vi "MV3D RGBD Set Param.vi"(9 "pstParam":T1={"enParamType"=1, "nReserved[0]"=0, "nReserved[1]"=0, "nReserved[2]"=0, "nReserved[3]"=0, "nReserved[4]"=0, "nReserved[5]"=0, "nReserved[6]"=0, "nReserved[7]"=0, "nReserved[8]"=0, "nReserved[9]"=0, "nReserved[10]"=0, "nReserved[11]"=0, "nReserved[12]"=0, "nReserved[13]"=0, "nReserved[14]"=0, "nReserved[15]"=0} {"enParamType" items=["ParamType_Bool"=1, "ParamType_Int"=2, "ParamType_Float"=3, "ParamType_Enum"=4, "ParamType_String"=5]}, 10 "strKey":string, 11 "handle":u32) -> (1 "pstParam out":T1={"enParamType"=1, "nReserved[0]"=0, "nReserved[1]"=0, "nReserved[2]"=0, "nReserved[3]"=0, "nReserved[4]"=0, "nReserved[5]"=0, "nReserved[6]"=0, "nReserved[7]"=0, "nReserved[8]"=0, "nReserved[9]"=0, "nReserved[10]"=0, "nReserved[11]"=0, "nReserved[12]"=0, "nReserved[13]"=0, "nReserved[14]"=0, "nReserved[15]"=0} {"enParamType" items=["ParamType_Bool"=1, "ParamType_Int"=2, "ParamType_Float"=3, "ParamType_Enum"=4, "ParamType_String"=5]}, 2 "function return":i32, 3 "handle out":u32)   [LabVIEW 2015, in "Mv3dRgbd.lvlib"]
doc: "MV3D_RGBD_API MV3D_RGBD_STATUS MV3D_RGBD_SetParam(HANDLE handle, const char* strKey, MV3D_RGBD_PARAM* pstParam);"
uses:
  <userlib>/Mv3dRgbd/Mv3dRgbd.lvlib
  <userlib>/Mv3dRgbd/Mv3dRgbd.dll
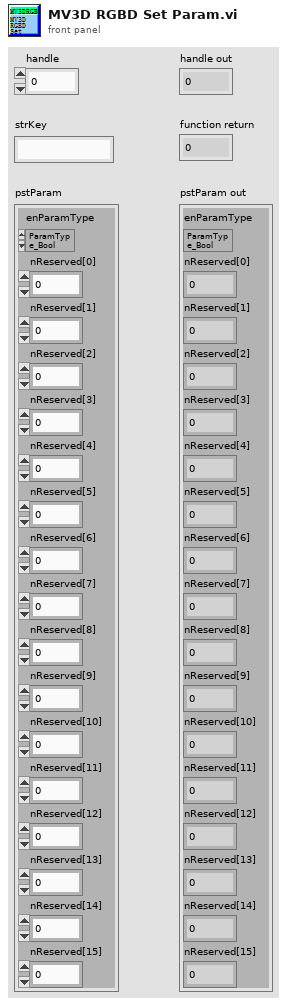
[diagram p1: front panel]
types:
  T1 = cluster{"enParamType":u32, "nReserved[0]":u8, "nReserved[1]":u8, "nReserved[2]":u8, "nReserved[3]":u8, "nReserved[4]":u8, "nReserved[5]":u8, "nReserved[6]":u8, "nReserved[7]":u8, "nReserved[8]":u8, "nReserved[9]":u8, "nReserved[10]":u8, "nReserved[11]":u8, "nReserved[12]":u8, "nReserved[13]":u8, "nReserved[14]":u8, "nReserved[15]":u8}
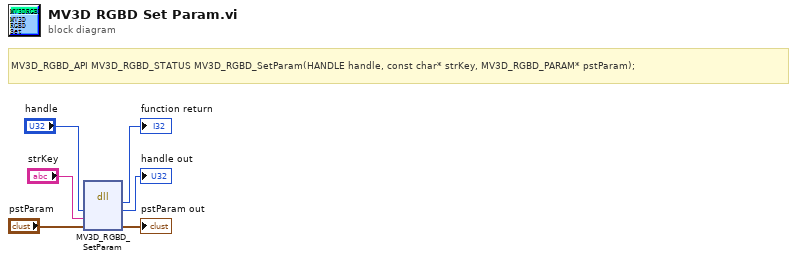
[diagram p0: block diagram]
diagram:
  # "MV3D_RGBD_API MV3D_RGBD_STATUS MV3D_RGBD_SetParam(HANDLE handle, const char* strKey, MV3D_RGBD_PARAM* pstParam);"
  n1 = dll-call lib="C:/Program Files (x86)/National Instruments/LabVIEW 2015/user.lib/Mv3dRgbd/Mv3dRgbd.*" fn="MV3D_RGBD_SetParam"("handle"="handle", "strKey"="strKey", "pstParam"="pstParam") -> (→"function return":i32, "handle"=→"handle out":u32, "pstParam"=→"pstParam out":T1)  [unwired: 4 in, 2 out]
